vi "Nema 2 spreadsheet string.vi"(6 "Grennich Offset":dbl, 9 "Antenna offset":dbl max=0.0, 10 "Nema string":string, 11 "RCVR":string) -> (3 "concatenated string":string)   [LabVIEW 2011]
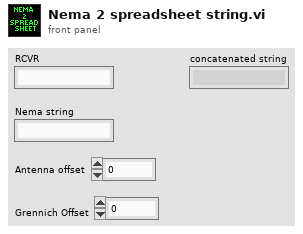
[diagram p1: front panel]
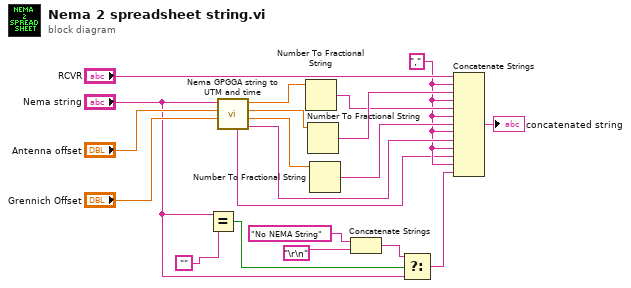
[diagram p0: block diagram]
diagram:
  w8 = "," ("string")
  n1 = Equal?(x="Nema string", y="") -> (x = y?=w5:bool)
  n2 = call "Nema GPGGA string to UTM and time.vi"("Grennich Offset"="Grennich Offset", "Antenna offset"="Antenna offset", "String In (NEAMA GGA)"="Nema string") -> ("date/time string"=w9:string, "Elevation"=w11:dbl, "Easting (M)"=w12:dbl, "Northing (M)"=w13:dbl, "Zone (string)"=w7:string)  [unwired: 4 in]
  n3 = Number To Fractional String(number=w13) -> (F-format string=w14:string)  [unwired: 3 in]
  n4 = Number To Fractional String(number=w12) -> (F-format string=w15:string)  [unwired: 3 in]
  n5 = Number To Fractional String(number=w11) -> (F-format string=w10:string)  [unwired: 3 in]
  n6 = Concatenate Strings("No NEMA String" ("string"), "\r\n") -> (w2:string)
  n7 = Select(t=w2, s=w5, f="Nema string") -> (s? t:f=w4:string)
  n8 = Concatenate Strings("RCVR", w8, w15, w8, w14, w8, w10, w8, w9, w8, w7, w8, w4) -> (→"concatenated string":string)
